vi "PB_add_VLIW.vi"(0 "VLIW Array In":T1(array[cluster]) {"OP Code" format="%.0x"; "Output Bits" format="%.0x"}, 1 "Data Field":u32, 2 "Digital Bits":u32 format="%.0x", 3 "Delay":dbl=50.0 format="%.3p", 4 "OP code":u8(ring) items=["Continue", "Stop", "Loop", "End Loop", "Jump", "Return", "Go To", "Long Delay", "Wait"], 5 "error in (no error)":errorcluster) -> (6 "VLIW Array Out":T1(array[cluster])=[{"Output Bits"=0, "Data Field"=3, "OP Code"=2, "Delay Count"=4}, {"Output Bits"=0, "Data Field"=0, "OP Code"=3, "Delay Count"=4}, {"Output Bits"=0, "Data Field"=0, "OP Code"=0, "Delay Count"=2599999997}, {"Output Bits"=0, "Data Field"=2, "OP Code"=7, "Delay Count"=1073741821}, {"Output Bits"=0, "Data Field"=0, "OP Code"=0, "Delay Count"=705032701}] {"OP Code" format="%.0x"; "Output Bits" format="%.0x"}, 7 "Actual Delay":dbl=50.0 format="%.2p", 8 "error out":errorcluster)   [LabVIEW 2013, in "PulseBlaster.lvlib"]
doc: "This vi writes a single command to \"VLIW Array\", where \"VLIW array\" is an array of clusters which contain an image of the command array of the PulseBlaster.\n\nIt provides some error checking on the inputs to help make sure you won't confuse the PulseBlaster.\nInputs:\n 1) Digital Bits (24 bit output flags)\n 2) Data Field (24 bits)\n 3) OP Code (4 bits)\n 4) Delay (in units of seconds)\n 5) error in.\n 6) Input array (The array to be appended to.)\nOutputs\n 1) Actual Delay (in units of seconds, rounded to nearest 10ns)\n 2) error out.\n 3) Output array. (The appended array.)\n\n\"PB_add_VLIW\" uses the globally defined variables in \"PB_defines\". The long delay command should be entirely transparent, so the user does not need to envoke it."
uses:
  PulseBlaster.lvlib
  PB_defines.vi
panel:
  # "append"
  # "to"
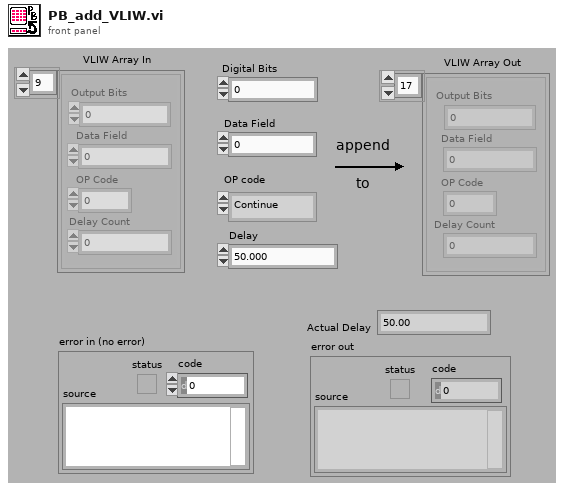
[diagram p1: front panel]
types:
  T1 = cluster{"Output Bits":u32, "Data Field":u32, "OP Code":u8, "Delay Count":u64}[]
  T2 = cluster{"Output Bits":u32, "Data Field":u32, "OP Code":u8, "Delay Count":u64}
  T3 = cluster{"Digital Bits":u32, "Data Field":u32, "OP code":u8, u64}
  T4 = cluster{"Digital Bits":u32, "Data Field":u32, "OP code":u8, "Delay Count":u64}[]
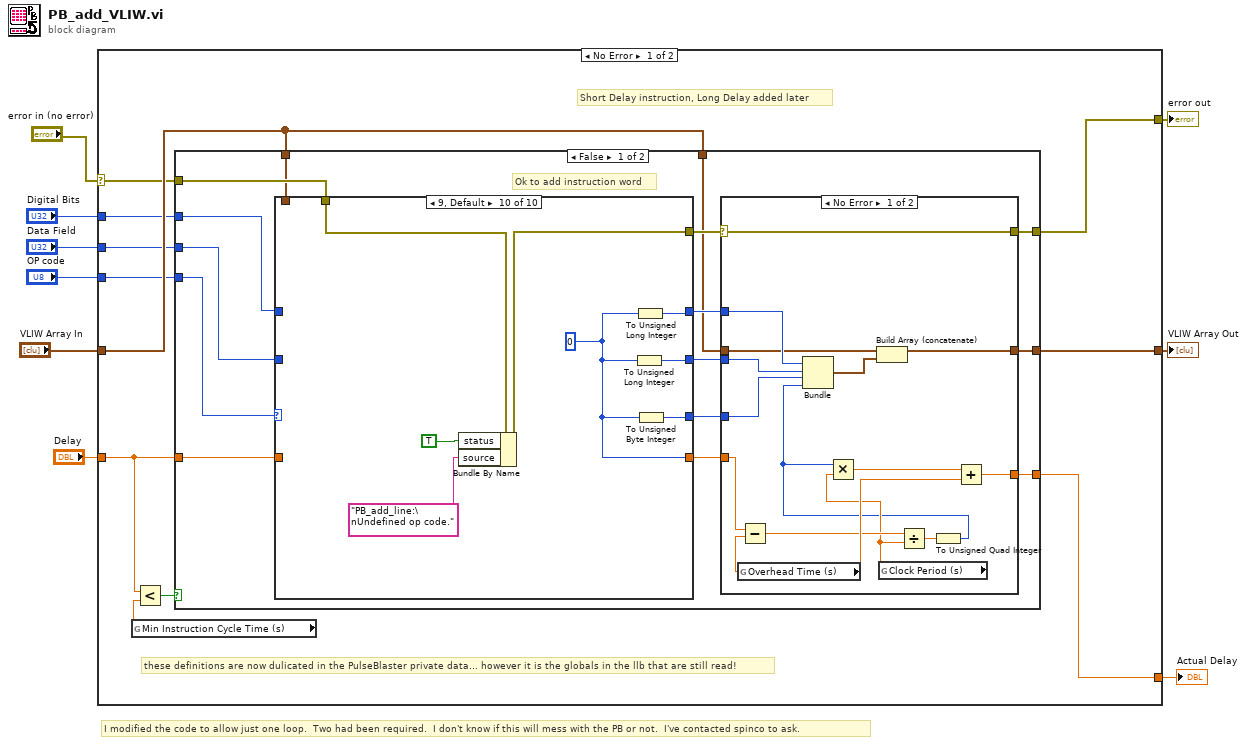
[diagram p0: block diagram]
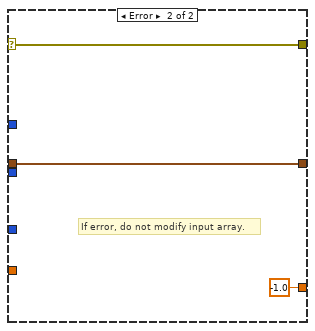
[diagram p2: hidden frame]
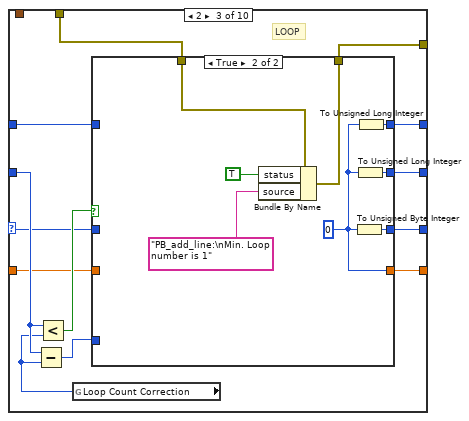
[diagram p5: hidden frame]
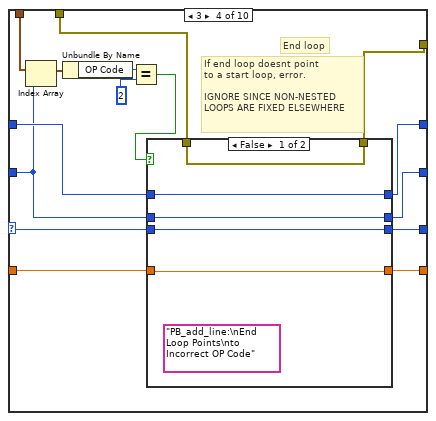
[diagram p7: hidden frame]
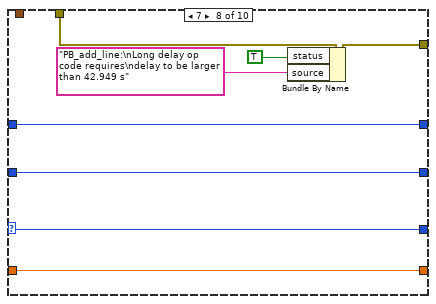
[diagram p12: hidden frame]
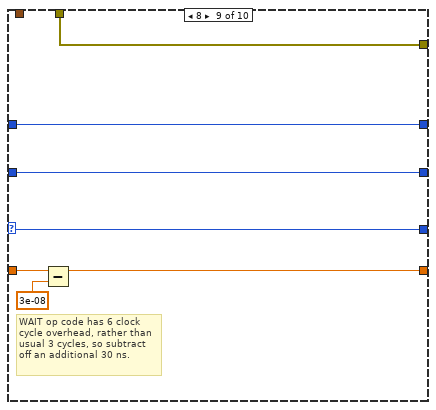
[diagram p13: hidden frame]
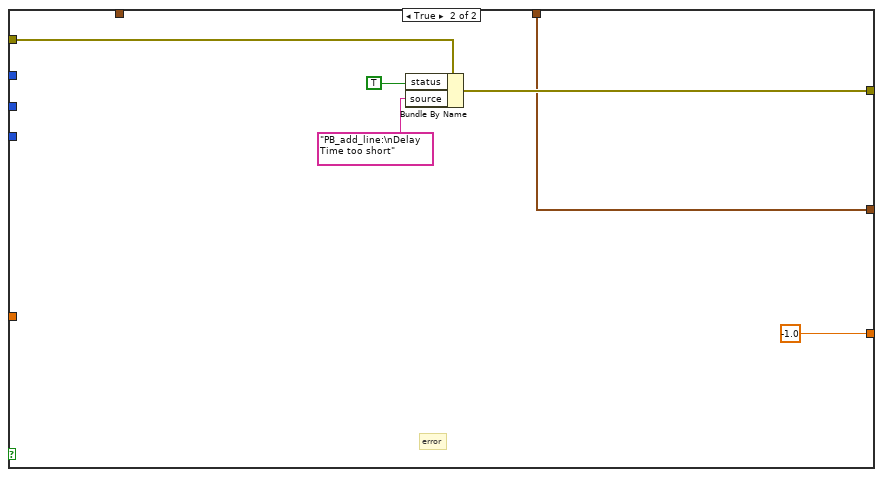
[diagram p14: hidden frame]
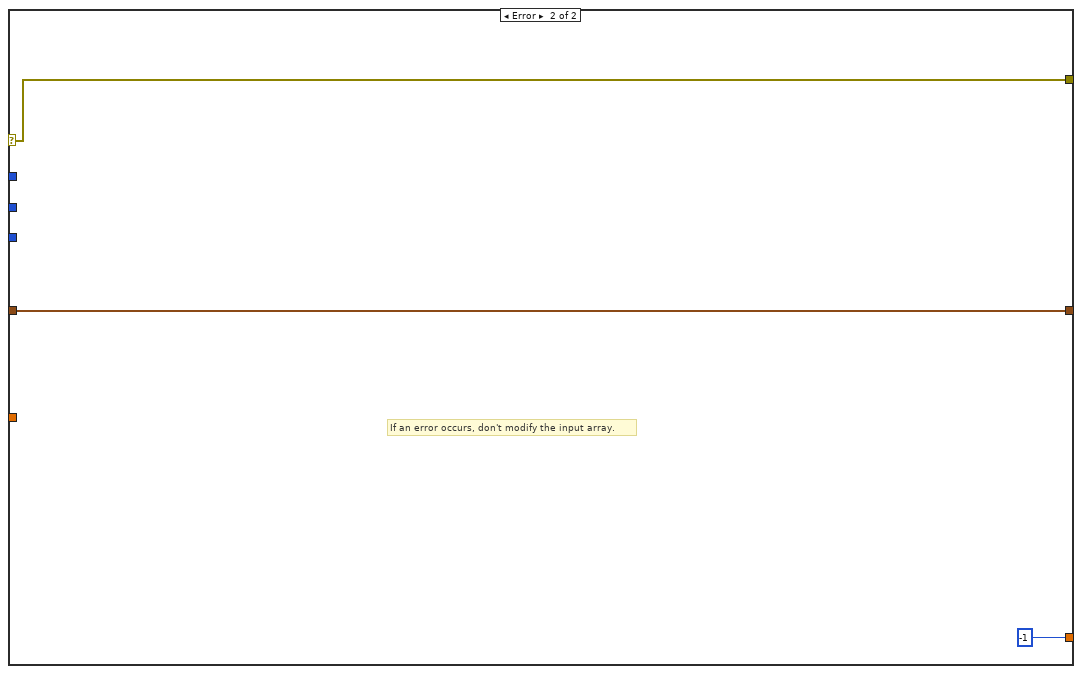
[diagram p15: hidden frame]
diagram:
  # "I modified the code to allow just one loop.  Two had been required.  I don't know if this will mess with the PB or not.  I've contacted spinco to ask."
  n1 = case shown="No Error" "error in (no error)" {
    selector: "error in (no error)" -> [w10 w159]
    tunnel: [w20 w159] -> w9
    tunnel: [w19 -1] -> w7
    tunnel: [w18 w160] -> w6
    tunnel: "VLIW Array In" -> [w17 w160]
    tunnel: "Digital Bits" -> [w16 _]
    tunnel: "Data Field" -> [w15 _]
    tunnel: "OP code" -> [w14 _]
    tunnel: "Delay" -> [w11 _]
    frame No Error {
      # "these definitions are now dulicated in the PulseBlaster private data... however it is the globals in the llb that are still read!"
      # "Short Delay instruction, Long Delay added later"
      n2 = global read "PB_defines.vi" "Min Instruction Cycle Time (s)"() -> (w13:dbl)
      n3 = Less?(x=w11, y=w13) -> (x < y?=w12:bool)
      n4 = case shown="False" w12 {
        tunnel: w10 -> [w35 w158]
        tunnel: [w34 w157] -> w20
        tunnel: [w28 -1.0] -> w19
        tunnel: w11 -> [w27 _]
        tunnel: [w26 w154] -> w18
        tunnel: w17 -> [w25 w154]
        tunnel: w16 -> [w24 _]
        tunnel: w15 -> [w23 _]
        tunnel: w14 -> [w22 _]
        tunnel: w17 -> [w21 _]
        frame False {
          # "Ok to add instruction word"
          n5 = case shown="9, Default" w22 {
            selector: w22 -> [w54 w59 w64 w90 w115 w120 w125 w130 w138 _]
            tunnel: w35 -> [w58 w60 w73 w101 w119 w121 w126 w136 w144 w149]
            tunnel: [w58 w60 w72 w102 w119 w121 w126 w135 w144 w150] -> w29
            tunnel: [w57 w63 w71 w97 w118 w124 w129 w134 w143 w146] -> w33
            tunnel: w24 -> [w57 w63 w67 w100 w118 w124 w129 w134 w143 _]
            tunnel: [w56 w62 w70 w96 w117 w123 w128 w133 w142 w145] -> w32
            tunnel: w23 -> [w56 w62 w76 w99 w117 w123 w128 w133 w142 _]
            tunnel: [w54 w59 w69 w95 w115 w120 w125 w130 w138 w147] -> w31
            tunnel: [w55 w61 w68 w94 w116 w122 w127 w132 w139 w148] -> w30
            tunnel: w27 -> [w55 w61 w66 w98 w116 w122 w127 w132 w140 _]
            tunnel: w21 -> [_ _ _ w91 _ _ _ _ _ _]
            frame 0 {
              # "Continue"
            }
            frame 1 {
              # "Stop"
            }
            frame 2 {
              # "LOOP"
              n6 = global read "PB_defines.vi" "Loop Count Correction"() -> (w75:u8)
              n7 = Subtract(x=w76, y=w75) -> (x-y=w65:u32)
              n8 = Less?(x=w76, y=w75) -> (x < y?=w74:bool)
              n9 = case shown="True" w74 {
                tunnel: w73 -> [w81 w87]
                tunnel: [w81 w86] -> w72
                tunnel: [w80 w82] -> w71
                tunnel: [w79 w83] -> w70
                tunnel: [w77 w84] -> w69
                tunnel: [w78 w85] -> w68
                tunnel: w67 -> [w80 _]
                tunnel: w65 -> [w79 _]
                tunnel: w66 -> [w78 _]
                tunnel: w64 -> [w77 _]
                frame False {
                }
                frame True {
                  w85 = 0
                  n10 = Bundle By Name(cluster=w87, "status"=TRUE, "source"="PB_add_line:\nMin. Loop number is 1") -> (w86:errorcluster)
                  n11 = To Unsigned Byte Integer(number=w85) -> (unsigned 8bit integer=w84:u8)
                  n12 = To Unsigned Long Integer(number=w85) -> (unsigned 32bit integer=w83:u32)
                  n13 = To Unsigned Long Integer(number=w85) -> (unsigned 32bit integer=w82:u32)
                }
              }
            }
            frame 3 {
              # "If end loop doesnt point\nto a start loop, error.\n\nIGNORE SINCE NON-NESTED\nLOOPS ARE FIXED ELSEWHERE"
              # "End loop"
              n14 = Index Array(array=w91, index=w99) -> (element=w93:T2)
              n15 = Unbundle By Name(w93) -> ("OP Code"=w92:u8)
              n16 = Equal?(x=w92, y=2) -> (x = y?=w103:bool)
              n17 = case shown="False" w103 {
                tunnel: [w105 w114] -> w102
                tunnel: w101 -> [w105 w114]
                tunnel: w100 -> [w107 w112]
                tunnel: w99 -> [w109 w111]
                tunnel: [w109 w111] -> w96
                tunnel: w90 -> [w106 w110]
                tunnel: w98 -> [w108 w113]
                tunnel: [w108 w113] -> w94
                tunnel: [w107 w112] -> w97
                tunnel: [w106 w110] -> w95
                frame False {
                  (unwired) "PB_add_line:\nEnd Loop Points\nto Incorrect OP Code"
                }
                frame True {
                }
              }
            }
            frame 4 {
            }
            frame 5 {
            }
            frame 6 {
            }
            frame 7 {
              n18 = Bundle By Name(cluster=w136, "status"=TRUE, "source"="PB_add_line:\nLong delay op code requires\ndelay to be larger than 42.949 s") -> (w135:errorcluster)
            }
            frame 8 {
              # "WAIT op code has 6 clock\ncycle overhead, rather than\nusual 3 cycles, so subtract\noff an additional 30 ns."
              n19 = Subtract(x=w140, y=3e-08) -> (x-y=w139:dbl)
            }
            frame 9, Default {
              w148 = 0
              n20 = Bundle By Name(cluster=w149, "status"=TRUE, "source"="PB_add_line:\nUndefined op code.") -> (w150:errorcluster)
              n21 = To Unsigned Long Integer(number=w148) -> (unsigned 32bit integer=w145:u32)
              n22 = To Unsigned Long Integer(number=w148) -> (unsigned 32bit integer=w146:u32)
              n23 = To Unsigned Byte Integer(number=w148) -> (unsigned 8bit integer=w147:u8)
            }
          }
          n24 = case shown="No Error" w29 {
            selector: w29 -> [w36 w51]
            tunnel: [w36 w51] -> w34
            tunnel: w33 -> [w43 _]
            tunnel: w32 -> [w44 _]
            tunnel: w31 -> [w45 _]
            tunnel: w30 -> [w46 _]
            tunnel: [w39 -1.0] -> w28
            tunnel: [w38 w52] -> w26
            tunnel: w25 -> [w37 w52]
            frame No Error {
              n25 = global read "PB_defines.vi" "Overhead Time (s)"() -> (w50:dbl)
              n26 = Subtract(x=w46, y=w50) -> (x-y=w49:dbl)
              n27 = global read "PB_defines.vi" "Clock Period (s)"() -> (w48:dbl)
              n28 = Divide(x=w49, y=w48) -> (x/y=w47:dbl)
              n29 = To Unsigned Quad Integer(1:w47) -> (0:w41:u64)
              n30 = Bundle("Digital Bits"=w43, "Data Field"=w44, "OP code"=w45, w41) -> (w42:T3)  [unwired: 1 out]
              n31 = Multiply(x=w41, y=w48) -> (x*y=w40:dbl)
              n32 = Build Array (concatenate)(w37, w42) -> (w38:T4)
              n33 = Add(x=w40, y=w50) -> (x+y=w39:dbl)
            }
            frame Error {
              # "If error, do not modify input array."
            }
          }
        }
        frame True {
          # "error"
          n34 = Bundle By Name(cluster=w158, "status"=TRUE, "source"="PB_add_line:\nDelay Time too short") -> (w157:errorcluster)
        }
      }
    }
    frame Error {
      # "If an error occurs, don't modify the input array."
    }
  }
  "error out" <- w9
  "Actual Delay" <- w7
  "VLIW Array Out" <- w6
